vi "ProdaNG.Tree.Results.TestValues.Add.vi"(6 "TestStepResultIDs":string[](array[string]), 7 "TestStepsTree":refnum<vi>, 8 "error in (no error)":errorcluster, 9 "units":T1[](array[typedef]), 10 "testStepId":i32, 11 "dbHandleIn":i32) -> (0 "error out":errorcluster, 3 "dbHandle":i32)   [LabVIEW 2016]
doc: "This function returns a product structure for a product, which is identified by a part and a serial number.\nImportant information: The field 'individual' was taken over from the field 'allgemein' of the legacy data directly. Because of this most products have the value 0 further on and only a few the value 1. \nParameter:\nhandle is an Integer, which is returned by the function Login() at the creation of a new connection.\nwabcoPartId is the Id of the part.\nserialNumber is the serial number of the product for the part above.\nproduct is a pointer on a product structure, which is filled if the returncode is 0. The structure must be defined in the calling program.\n\nReturncodes:\n0 No error\n< 0 ORACLE Error code\n6 (ERROR_INVALID_HANDLE) in case of an invalid handle\n1403 Record does not exist"
uses:
  Controls/ProdaNG.UnitSimple.ctl
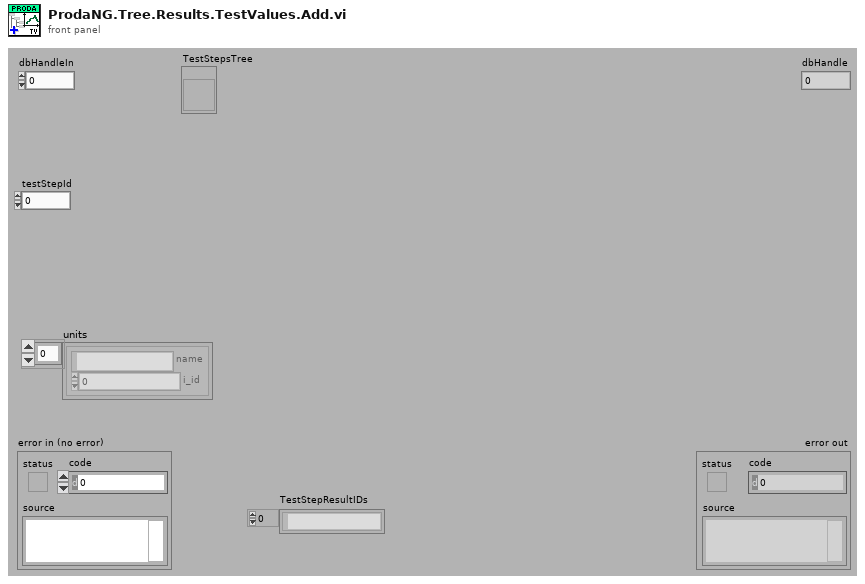
[diagram p1: front panel]
types:
  T1 = typedef "ProdaNG.UnitSimple.ctl" = cluster{"name":string, "i_id":i32}
  T2 = typedef "ProdaNG.TestValue.ctl" = cluster{"i_id":i32, "testStepId":i32, "releaseId":i32, "unitId":i32, "contentId":string, "previewId":string, "maximum":dbl, "minimum":dbl, "valueText":string, "testValueSequence":i32, "history":i32, "mdReason":string, "mdUser":string, "mdTime":string, "description":string}
  T3 = typedef "ProdaNG.TestValueResult.ctl" = cluster{"c_id":string, "testStepResultId":string, "testValueId":i32, "result":dbl, "statusId":i32, "contentId":string}
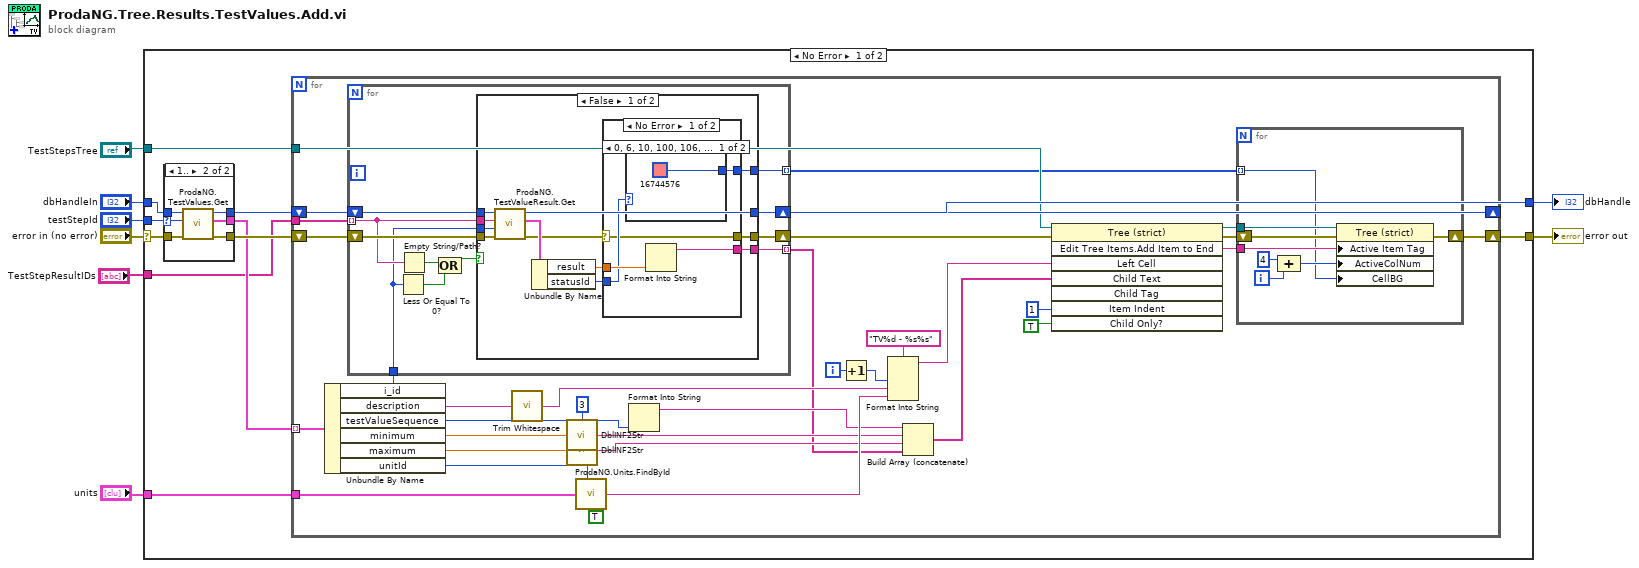
[diagram p0: block diagram]
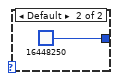
[diagram p3: hidden frame]
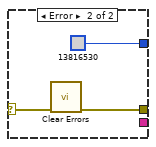
[diagram p4: hidden frame]
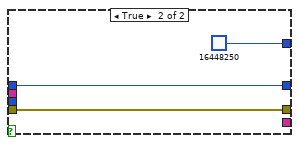
[diagram p5: hidden frame]
diagram:
  n1 = case shown="No Error" "error in (no error)" {
    selector: "error in (no error)" -> [w18 w106]
    tunnel: [w11 w106] -> w5
    tunnel: "dbHandleIn" -> [w17 w105]
    tunnel: [w10 w105] -> w4
    tunnel: "testStepId" -> [w12 _]
    tunnel: "TestStepsTree" -> [w15 _]
    tunnel: "units" -> [w14 _]
    tunnel: "TestStepResultIDs" -> [w9 _]
    frame No Error {
      n2 = case shown="1.." w12 {
        selector: w12 -> [_ w21]
        tunnel: w18 -> [w19 w26]
        tunnel: w17 -> [w20 w25]
        tunnel: [w20 w24] -> w10
        tunnel: [w19 w23] -> w16
        tunnel: [_ w22] -> w13
        frame Default {
        }
        frame 1.. {
          n3 = call "ProdaNG.TestValues.Get.vi"("error in (no error)"=w26, "testStepId"=w21, "dbHandleIn"=w25) -> ("error out"=w23:errorcluster, "TestStepValues"=w22:T2[], "dbHandle"=w24:i32)  [unwired: 6 in]
        }
      }
      n4 = for {
        shift-right: [w30] -> w11
        shift-left: w16 -> [w41]
        tunnel: w13 -> [w59] mode=indexing
        tunnel: w15 -> [w37]
        tunnel: w14 -> [w55]
        shift-right: [w39] -> _
        shift-left: w10 -> [w40]
        tunnel: w9 -> [w36]
        i -> [w57]
        w51 = i16 3 ("precision (6)")
        n5 = Unbundle By Name(w59) -> ("i_id"=w35:i32, "description"=w58:string, "testValueSequence"=w48:i32, "minimum"=w52:dbl, "maximum"=w53:dbl, "unitId"=w56:i32)
        n6 = for {
          shift-right: [w64] -> w38
          shift-left: w41 -> [w71]
          shift-right: [w69] -> w39
          shift-left: w40 -> [w70]
          tunnel: w36 -> [w68] mode=indexing
          tunnel: w35 -> [w63]
          tunnel: [w62] -> w34 mode=indexing
          tunnel: [w61] -> w28 mode=indexing
          n7 = Less Or Equal To 0?(x=w63) -> (x <= 0?=w66:bool)
          n8 = Empty String/Path?(string/path=w68) -> (empty?=w67:bool)
          n9 = Compound Arithmetic op=OR(w67, w66) -> (w65:bool)
          n10 = case shown="False" w65 {
            tunnel: w71 -> [w83 w95]
            tunnel: w70 -> [w82 w96]
            tunnel: [w81 w96] -> w69
            tunnel: w68 -> [w80 _]
            tunnel: [w73 w95] -> w64
            tunnel: w63 -> [w79 _]
            tunnel: [w76 _] -> w62
            tunnel: [w75 u32 16448250] -> w61
            frame False {
              n11 = call "ProdaNG.TestValueResult.Get.vi"("error in (no error)"=w83, "testValueId"=w79, "testStepResultId"=w80, "dbHandle"=w82) -> ("error out"=w74:errorcluster, "TestValueResult"=w77:T3, "dbHandle"=w81:i32)  [unwired: 5 in]
              n12 = Unbundle By Name(w77) -> ("result"=w78:dbl, "statusId"=w72:i32)
              n13 = case shown="No Error" w74 {
                selector: w74 -> [w84 w93]
                tunnel: w78 -> [w88 _]
                tunnel: [w87 _] -> w76
                tunnel: [w86 u32 13816530] -> w75
                tunnel: [w84 w92] -> w73
                tunnel: w72 -> [w85 _]
                frame No Error {
                  n14 = case shown="0, 6, 10, 100, 106, 110" w85 {
                    tunnel: [u32 16744576 u32 16448250] -> w86
                    frame 0, 6, 10, 100, 106, 110 {
                    }
                    frame Default {
                    }
                  }
                  n15 = Format Into String(w88) -> (resulting string=w87:string)  [unwired: 3 in, 1 out]
                }
                frame Error {
                  n16 = call <vilib>:"Clear Errors.vi"("error in (no error)"=w93) -> ("error out"=w92:errorcluster)  [unwired: 5 in, 1 out]
                }
              }
            }
            frame True {
            }
          }
        }
        n17 = call <vilib>:"Trim Whitespace.vi"("string"=w58) -> ("trimmed string"=w47:string)  [unwired: 1 in]
        n18 = call "DblINF2Str.vi"("Numeric"=w52, "precision (6)"=w51) -> ("string"=w49:string)
        n19 = call "DblINF2Str.vi"("Numeric"=w53, "precision (6)"=w51) -> ("string"=w46:string)
        n20 = call "ProdaNG.Units.FindById.vi"("units"=w55, "unit id"=w56, "add brackets (F)"=TRUE ("add quotas (F)")) -> ("unit str"=w54:string)
        n21 = Format Into String(w48) -> (resulting string=w45:string)  [unwired: 3 in, 1 out]
        n22 = Increment(x=w57) -> (x+1=w60:i32)
        n23 = Format Into String(format string="TV%d - %s%s", w60, w47, w54) -> (resulting string=w44:string)  [unwired: 2 in, 1 out]
        n24 = Build Array (concatenate)(w45, w49, w46, w34) -> (w43:string[])
        n25 = invoke on="Invoke Node" class="Tree (strict)" method="Edit Tree Items.Add Item to End"(reference=w37, error in=w38, "Left Cell"=w44, "Child Text"=w43, "Item Indent"=1 ("New Item Indentation"), "Child Only?"=TRUE) -> (reference out=w29:refnum<vi>, error out=w31:errorcluster, "Edit Tree Items:Add Item to End"=w27:string)  [unwired: 2 in, 5 out]
        n26 = for {
          tunnel: w29 -> [w104]
          tunnel: w27 -> [w101]
          shift-right: [w103] -> w30
          shift-left: w31 -> [w102]
          tunnel: w28 -> [w99] mode=indexing
          i -> [w97]
          n27 = Compound Arithmetic op=ADD(4 ("value"), w97) -> (w100:i32)
          n28 = property class="Tree (strict)"(reference=w104, error in=w102, "Active Item Tag"=w101, "ActiveColNum"=w100, "CellBG"=w99) -> (error out=w103:errorcluster)  [unwired: 1 out]
        }
      }
    }
    frame Error {
    }
  }
  "error out" <- w5
  "dbHandle" <- w4
